vi "item distribution.vi"(7 "original items":u32[](array[numeric]), 9 "item distributed":u32) -> (1 "item":u32[](array[numeric]))   [LabVIEW 2025]
panel:
  out "Numeric 2":i32
  out "Boolean":bool
  out "Numeric":i32
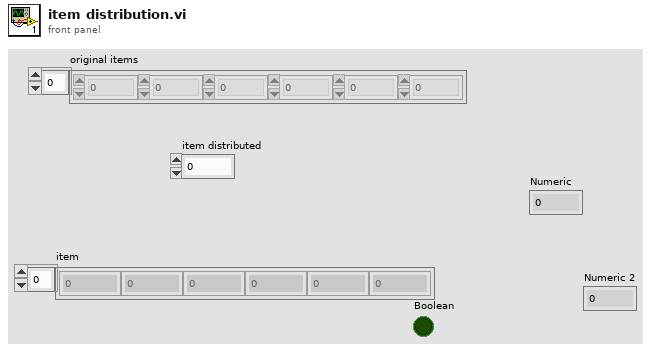
[diagram p1: front panel]
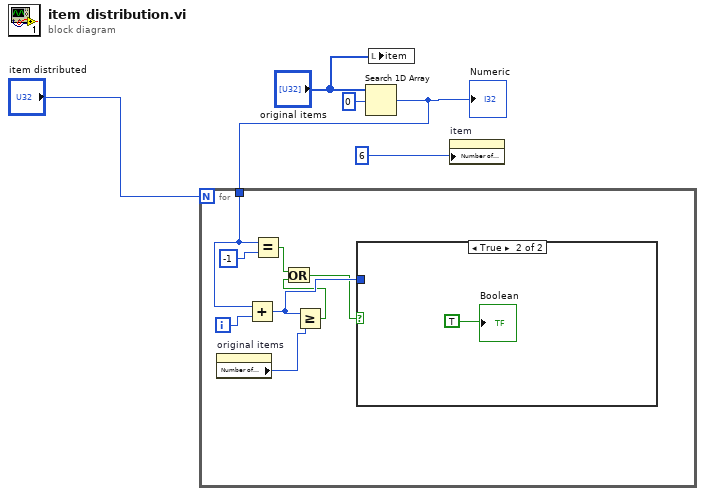
[diagram p0: block diagram]
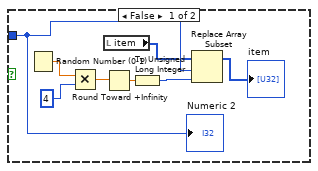
[diagram p2: hidden frame]
diagram:
  n1 = Search 1D Array(1D array="original items", element=u32 0) -> (index of element=w3:i32)  [unwired: 1 in]
  "Numeric" <- w3
  n2 = for {
    N: "item distributed" -> [_]
    tunnel: w3 -> [w10]
    i -> [w11]
    n3 = property on="original items" class="Arr (strict)"() -> ("Number of Columns"=w9:u32)  [unwired: 2 in, 2 out]
    n4 = Add(x=w10, y=w11) -> (x+y=w8:i32)
    n5 = Equal?(x=w10, y=-1) -> (x = y?=w12:bool)
    n6 = Greater Or Equal?(x=w8, y=w9) -> (x >= y?=w7:bool)
    n7 = Or(x=w12, y=w7) -> (x .or. y?=w6:bool)
    n8 = case shown="True" w6 {
      tunnel: w8 -> [w15 _]
      frame False {
        n9 = Random Number (0-1)() -> (number: 0 to 1=w21:dbl)
        n10 = Multiply(x=w21, y=4) -> (x*y=w20:dbl)
        n11 = local read "item"() -> (w14:u32[])
        n12 = Round Toward +Infinity(x=w20) -> (ceil(x): smallest int >= x=w19:dbl)
        n13 = To Unsigned Long Integer(number=w19) -> (unsigned 32bit integer=w17:u32)
        n14 = Replace Array Subset(array=w14, new element=w17, index=w15) -> (→"item":u32[])
        "Numeric 2" <- w15
      }
      frame True {
        "Boolean" <- TRUE
      }
    }
  }
  n15 = local write "item"("original items") -> ()
  n16 = property on="item" class="Arr (strict)"("Number of Columns"=u32 6) -> ()  [unwired: 2 in, 2 out]
